vi "solar_log Destroy.vi"(8 "error in (no error)":errorcluster) -> (0 "error out":errorcluster)   [LabVIEW 2018]
doc: "This destroys the logger process."
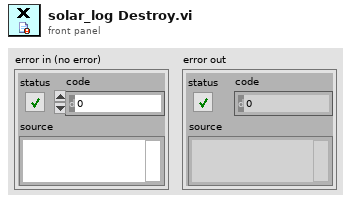
[diagram p1: front panel]
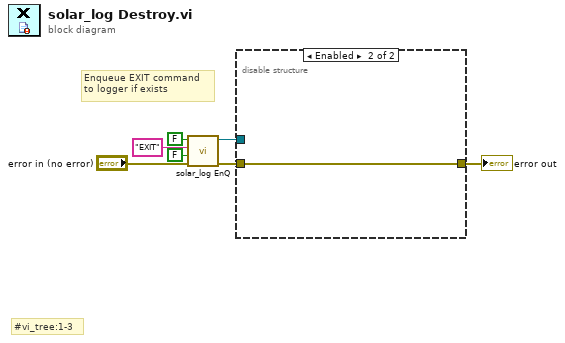
[diagram p0: block diagram]
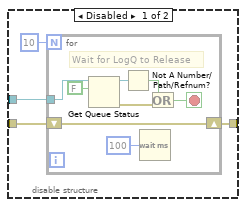
[diagram p2: hidden frame]
diagram:
  # "#vi_tree:1-3"
  # "Enqueue EXIT command\nto logger if exists"
  n1 = call "solar_log EnQ.vi"("error in (no error)"="error in (no error)", "Front? (F)"=FALSE, "MSG"="EXIT", "Create? (F)"=FALSE) -> ("error out"=w3:errorcluster, "LogQ"=w2:refnum<queue>)  [unwired: 5 in, 1 out]
  n2 = disable-structure shown="Enabled" {
    disable-tunnel: w3 -> [w11 w20]
    disable-tunnel: w2 -> [w10 _]
    disable-tunnel: [w8 w20] -> w1
    frame Disabled {
      n3 = for {
        N: 10 -> [_]
        tunnel: w10 -> [w19]
        shift-right: [w17] -> w8
        shift-left: w11 -> [w17]
        stop <- w15 stop-if-true
        # "Wait for LogQ to Release"
        n4 = Get Queue Status(queue=w19, return elements? (F)=FALSE) -> (queue out=w14:refnum<queue>, error out=w16:errorcluster)  [unwired: 1 in, 6 out]
        n5 = Not A Number/Path/Refnum?(number/path/refnum=w14) -> (NaN/Path/Refnum?=w13:bool)
        n6 = Wait (ms)(milliseconds to wait=u32 100) -> ()  [unwired: 1 out]
        n7 = Or(x=w13, y=w16) -> (x .or. y?=w15:bool)
      }
    }
    frame Enabled {
    }
  }
  "error out" <- w1
